vi "Explore_Volume.vi"(3 "Mode":T5, 5 "Traverse line In":T2 {"Row Duration (mins)" format="%#.1f"; "Row No" min=0; "Trace Gas Concentration (%)" min=0.0 format="%#.2f"; "Emission Rate (l/min)" format="%#.2f"; "Tunnel Speed" format="%#.2f"; "Start X" format="%#.2f"; "Start Y" format="%#.2f"; "Start Z" format="%#.2f"; "End X" format="%#.2f"; "End Y" format="%#.2f"; "End Z" format="%#.2f"; "Averaging time (min)" min=0.0 format="%#.2f"}) -> (0 "Error Message":string, 1 "Status":T1, 2 "Traverse line Out":T2 {"Row Duration (mins)" format="%#.1f"; "Row No" min=0; "Trace Gas Concentration (%)" min=0.0 format="%#.2f"; "Emission Rate (l/min)" format="%#.2f"; "Tunnel Speed" format="%#.2f"; "Start X" format="%#.2f"; "Start Y" format="%#.2f"; "Start Z" format="%#.2f"; "End X" format="%#.2f"; "End Y" format="%#.2f"; "End Z" format="%#.2f"; "Averaging time (min)" min=0.0 format="%#.2f"})   [LabVIEW 2011]
uses:
  Gen Trav/Traverse_cluster.ctl
  Gen Trav/Spacing.ctl
  Controls/Multi_run_mode.ctl
  Controls/User_Specific_mode.ctl
  Gen Trav/Multi_Run_Status.ctl
  Controls/Save_Data.ctl
  Controls/Setup.ctl
panel:
  # "X           Y            Z"
  # "Start"
  # "End"
  # "X           Y            Z"
  # "Start"
  # "End"
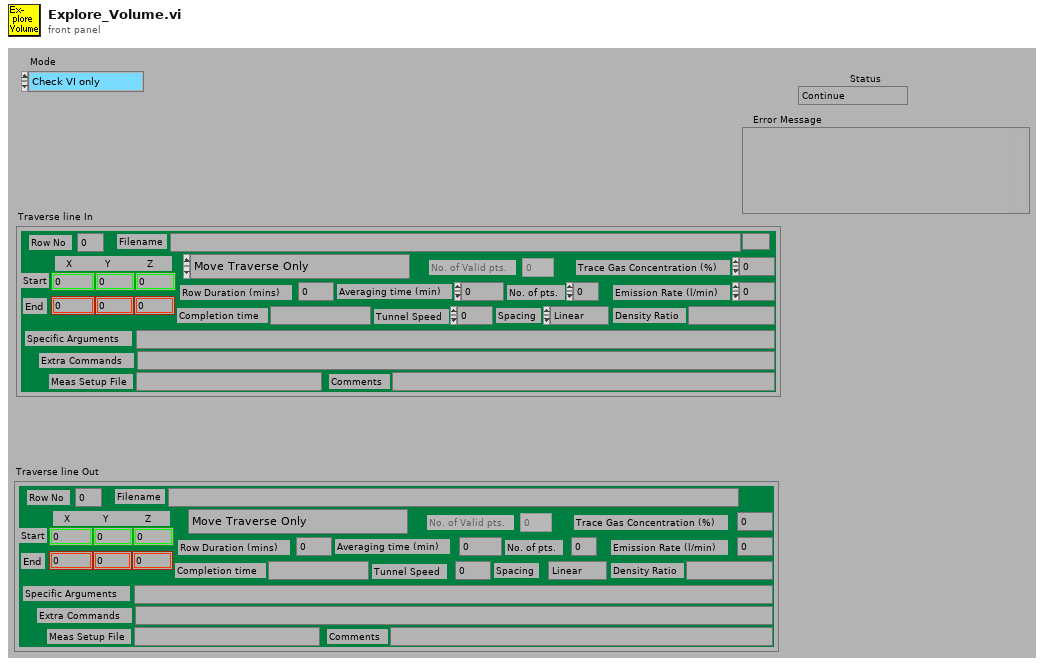
[diagram p1: front panel]
types:
  T1 = typedef "Multi_Run_Status.ctl" = enum16{"Continue", "Jump to Next Point", "Jump to Next Row", "Jump To Fall Back", "Terminate Run"}
  T2 = typedef "Traverse_cluster.ctl" = cluster{"Start X":dbl, "Start Y":dbl, "Start Z":dbl, "End X":dbl, "End Y":dbl, "End Z":dbl, "No. of pts.":i32, "Spacing":T3, "Filename":path, "Tunnel Speed":dbl, "Averaging time (min)":dbl, "Extra Commands":string, "Specific Arguments":string, "Emission Rate (l/min)":dbl, "Trace Gas Concentration (%)":dbl, "Density Ratio":string, "Comments":string, "Row No":i32, "Row Type Selector":T4, "Completion time":string, "Row Duration (mins)":dbl, "No. of Valid pts.":i32, "Meas Setup File":string}
  T3 = typedef "Spacing.ctl" = enum16{"Linear", "Log", "Gauss", "Specified", "N/A"}
  T4 = typedef "Multi_run_mode.ctl" = enum16{"Move Traverse Only", "Set Tunnel Speed Only", "Set Source Only", "Set Measurement Conditions", "Single Measurement", "Vertical Profile", "Lateral Profile", "Longitudinal Profile", "Explore Volume", "Multi-Axis Profile", "Auto Calibrate", "Meas Fast FID Bkgnd", "Check Beam Power", "Scanning Valve Measurement", "Run VI Named:", "Set ADAM Ch", "Wait (minutes)", "Send Message", "Synchronize With:", "Fall Back to this Row", "Turn Off Row Repeating", "Blank Row", "Traverse 3D Volume"}
  T5 = typedef "User_Specific_mode.ctl" = enum16{"Check VI only", "Run VI"}
  T6 = typedef "Save_Data.ctl" = enum16{"Save No Data", "Save Data"}
  T7 = typedef "Setup.ctl" = enum16{"Run Program", "Show Setup", "Save Current Setup", "Setup Front Panel"}
  T8 = typedef "Status_Cluster.ctl" = cluster{"Status":T1, "Error Type":string, "Error Description":string}
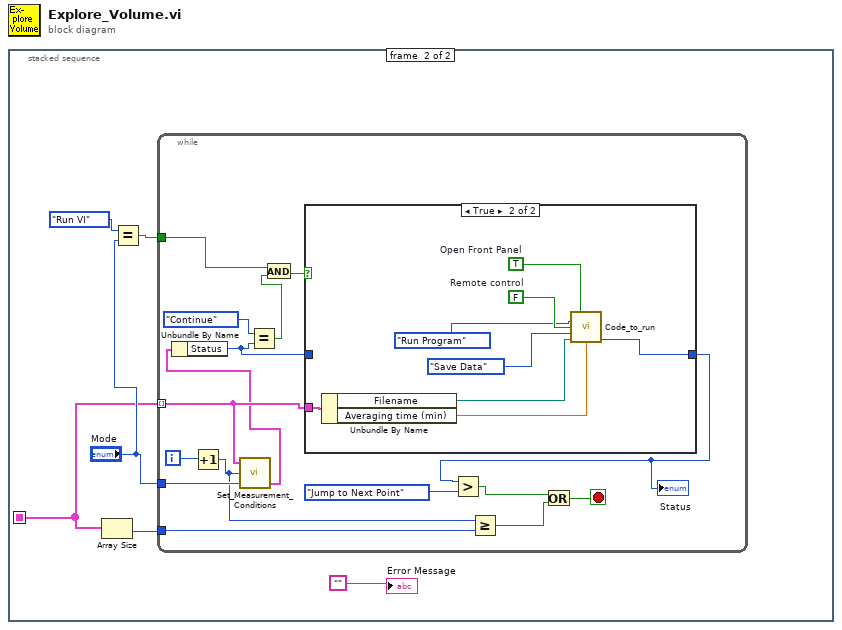
[diagram p0: block diagram]
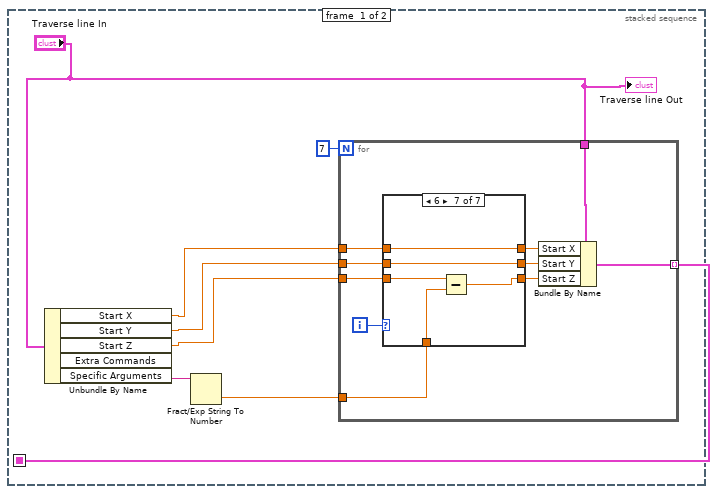
[diagram p2: hidden frame]
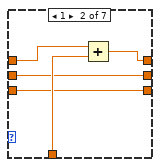
[diagram p4: hidden frame]
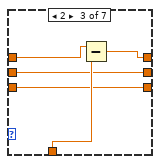
[diagram p5: hidden frame]
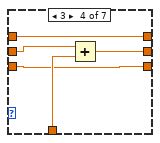
[diagram p6: hidden frame]
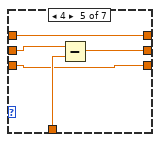
[diagram p7: hidden frame]
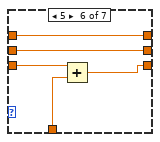
[diagram p8: hidden frame]
diagram:
  n1 = stacked-sequence {
    seq-local: [w2 _] -> [_ w54]
    frame #0 {
      n2 = Unbundle By Name("Traverse line In") -> ("Start X"=w6:dbl, "Start Y"=w5:dbl, "Start Z"=w4:dbl, "Specific Arguments"=w8:string)  [unwired: 1 out]
      n3 = Fract/Exp String To Number(string=w8) -> (number=w3:dbl)  [unwired: 3 in, 1 out]
      n4 = for {
        N: 7 -> [_]
        tunnel: "Traverse line In" -> [w18]
        tunnel: w6 -> [w16]
        tunnel: w5 -> [w14]
        tunnel: w4 -> [w12]
        tunnel: w3 -> [w10]
        tunnel: [w9] -> w2 mode=indexing
        i -> [w17]
        n5 = case shown="6" w17 {
          tunnel: w16 -> [w21 w25 w31 w34 w37 w42 w47]
          tunnel: [w21 w24 w30 w34 w37 w42 w47] -> w15
          tunnel: w14 -> [w20 w23 w28 w36 w41 w43 w48]
          tunnel: [w20 w23 w28 w32 w40 w43 w48] -> w13
          tunnel: w12 -> [w19 w22 w27 w33 w38 w46 w51]
          tunnel: [w19 w22 w27 w33 w38 w44 w49] -> w11
          tunnel: w10 -> [_ w26 w29 w35 w39 w45 w50]
          frame 0, Default {
          }
          frame 1 {
            n6 = Add(x=w25, y=w26) -> (x+y=w24:dbl)
          }
          frame 2 {
            n7 = Subtract(x=w31, y=w29) -> (x-y=w30:dbl)
          }
          frame 3 {
            n8 = Add(x=w36, y=w35) -> (x+y=w32:dbl)
          }
          frame 4 {
            n9 = Subtract(x=w41, y=w39) -> (x-y=w40:dbl)
          }
          frame 5 {
            n10 = Add(x=w46, y=w45) -> (x+y=w44:dbl)
          }
          frame 6 {
            n11 = Subtract(x=w51, y=w50) -> (x-y=w49:dbl)
          }
        }
        n12 = Bundle By Name(cluster=w18, "Start X"=w15, "Start Y"=w13, "Start Z"=w11) -> (w9:T2)
      }
      "Traverse line Out" <- "Traverse line In"
    }
    frame #1 {
      n13 = Array Size(array=w54) -> (size(s)=w53:i32)
      n14 = Equal?(x=User_Specific_mode."Run VI" ("Mode"), y="Mode") -> (x = y?=w55:bool)
      n15 = while {
        tunnel: w54 -> [w72] mode=indexing
        tunnel: "Mode" -> [w69]
        tunnel: w55 -> [w67]
        tunnel: w53 -> [w61]
        i -> [w73]
        stop <- w59 stop-if-true
        n16 = Increment(x=w73) -> (x+1=w62:i32)
        n17 = call "Set_Measurement_Conditions.vi"("Simulate/Run"=w69, "Currently on Point"=w62, "Traverse line"=w72) -> ("Status Cluster"=w71:T8)  [unwired: 2 in]
        n18 = Unbundle By Name(w71) -> ("Status"=w65:T1)
        n19 = Equal?(x=Multi_Run_Status."Continue" ("Status"), y=w65) -> (x = y?=w68:bool)
        n20 = And(x=w67, y=w68) -> (x .and. y?=w66:bool)
        n21 = case shown="True" w66 {
          tunnel: w72 -> [_ w82]
          tunnel: w65 -> [w74 _]
          tunnel: [w74 w76] -> w58
          frame False {
          }
          frame True {
            w79 = TRUE  # Open Front Panel
            w81 = FALSE  # Remote control
            n22 = Unbundle By Name(w82) -> ("Filename"=w75:path, "Averaging time (min)"=w80:dbl)
            n23 = call "Code_to_run.vi"("Open Front Panel"=w79, "setup"=Setup."Run Program", "Remote control"=w81, "File"=Save_Data."Save Data", "Results Filename"=w75, "Averaging time (min)"=w80) -> ("Status"=w76:T1)  [unwired: 9 in]
          }
        }
        "Status" <- w58
        n24 = Greater?(x=w58, y=Multi_Run_Status."Jump to Next Point" ("Status")) -> (0:w63:bool)
        n25 = Greater Or Equal?(x=w62, y=w61) -> (x >= y?=w60:bool)
        n26 = Or(x=w63, y=w60) -> (x .or. y?=w59:bool)
      }
      "Error Message" <- ""
    }
  }
